vi "NodoPropiedad.vi"() -> ()   [LabVIEW 2020]
panel:
  in  "Cadena de Caracteres":string
  in  "Boolean 2":bool
  in  "Posicion Horizontal":dbl(slide) scale=0.0..1000.0
  in  "Posicion Vertical":dbl(slide) scale=0.0..1000.0
  in  "Deshabilitar":bool
  in  "Limite":dbl
  in  "stop":bool
  out "Tank":dbl(slide) scale=0.0..10.0
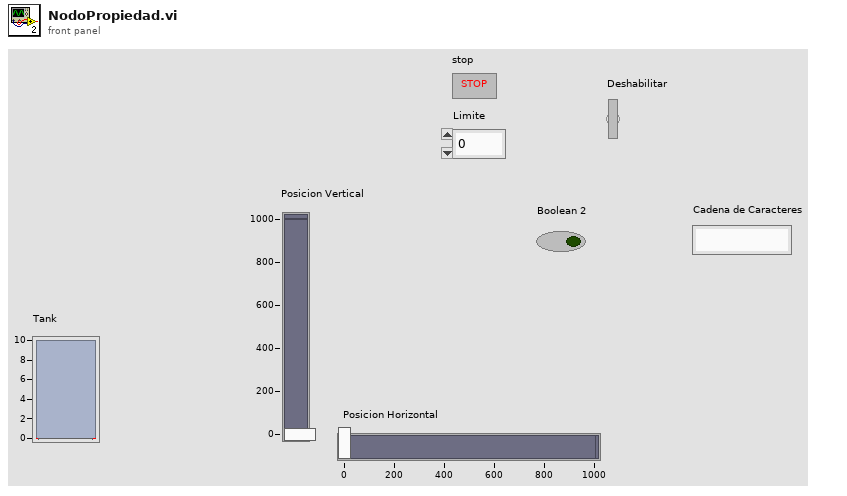
[diagram p1: front panel]
types:
  T1 = cluster{" Posicion Horizontal":dbl, "Posicion Vertical":dbl}
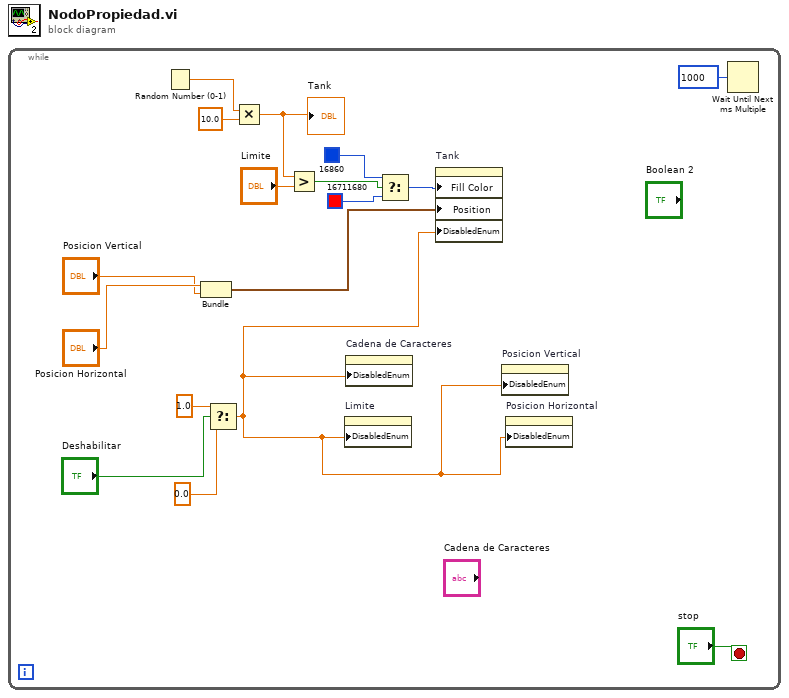
[diagram p0: block diagram]
diagram:
  n1 = while {
    stop <- "stop" stop-if-true
    n2 = Random Number (0-1)() -> (number: 0 to 1=w16:dbl)
    n3 = Bundle("Posicion Horizontal"="Posicion Horizontal", "Posicion Vertical"="Posicion Vertical") -> (w1:T1)  [unwired: 1 in]
    n4 = Select(t=1.0, s="Deshabilitar", f=0.0) -> (s? t:f=w4:dbl)
    n5 = Multiply(x=w16, y=10.0) -> (x*y=w14:dbl)
    "Tank" <- w14
    n6 = Greater?(x=w14, y="Limite") -> (0:w13:bool)
    n7 = property on="Limite" class="DigNum (strict)"("DisabledEnum"=w4) -> ()  [unwired: 2 in, 2 out]
    n8 = property on="Cadena de Caracteres" class="Str"("DisabledEnum"=w4) -> ()  [unwired: 2 in, 2 out]
    n9 = Select(t=u32 16860, s=w13, f=u32 16711680) -> (s? t:f=w8:u32)
    n10 = property on="Tank" class="Slide (strict)"("Fill Color"=w8, "Position"=w1, "DisabledEnum"=w4) -> ()  [unwired: 2 in, 2 out]
    n11 = property on="Posicion Vertical" class="Slide (strict)"("DisabledEnum"=w4) -> ()  [unwired: 2 in, 2 out]
    n12 = property on="Posicion Horizontal" class="Slide (strict)"("DisabledEnum"=w4) -> ()  [unwired: 2 in, 2 out]
    n13 = Wait Until Next ms Multiple(millisecond multiple=u32 1000) -> ()  [unwired: 1 out]
  }
